vi "Q-Close.vi"(8 "error in":errorcluster, 10 "Queue Type":T1, 11 "Q Name":string) -> (0 "error out":errorcluster)   [LabVIEW 2016]
uses:
  PSDAQEG_Task Queue Type.ctl
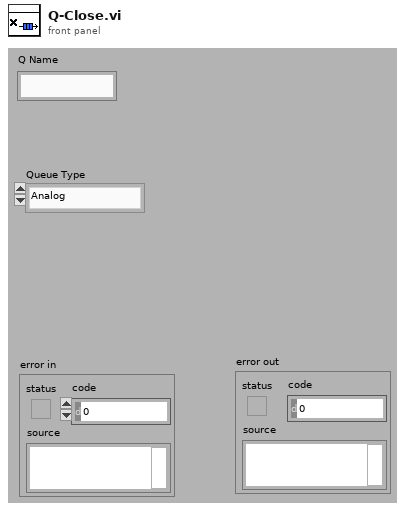
[diagram p1: front panel]
types:
  T1 = typedef "PSDAQEG_Task Queue Type.ctl" = enum16{"Analog", "Digital", "Variant"}
  T2 = cluster{"Analog Data":waveform(dbl)[], "Digital Data":digitalwaveform[], "Variant Data":variant[]}
  T3 = cluster{"max queue size (-1, unlimited)":i32, "Analog Data":waveform(dbl)[]}
  T4 = cluster{"max queue size (-1, unlimited)":i32, "Digital Data":digitalwaveform[]}
  T5 = cluster{"max queue size (-1, unlimited)":i32, "Variant Data":variant[]}
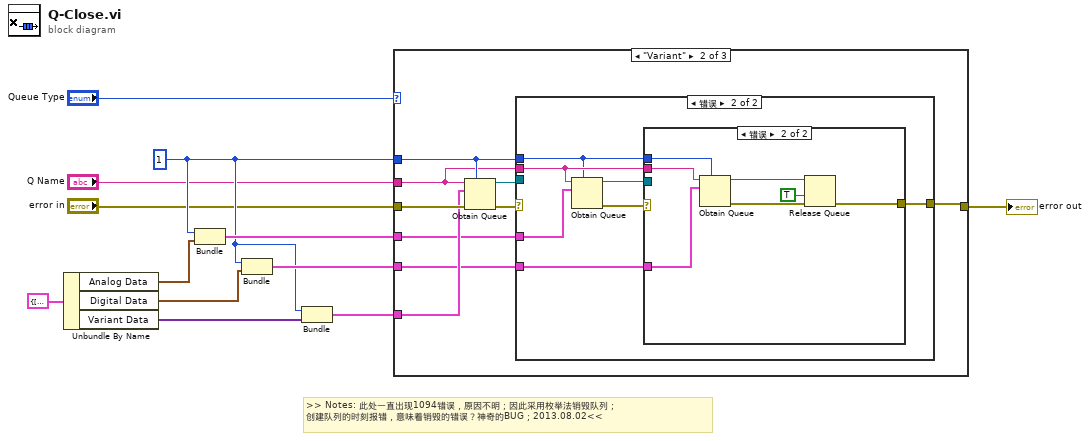
[diagram p0: block diagram]
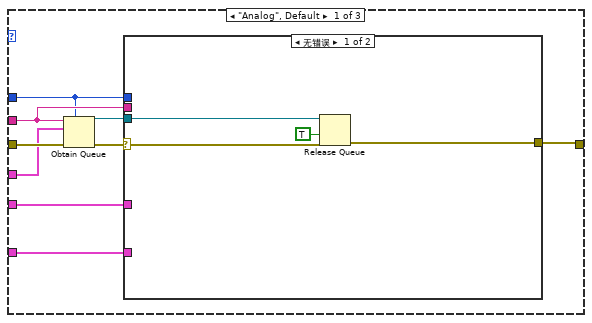
[diagram p2: hidden frame]
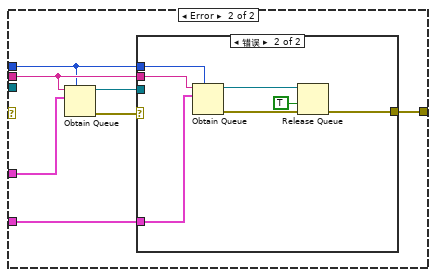
[diagram p3: hidden frame]
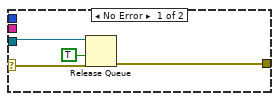
[diagram p4: hidden frame]
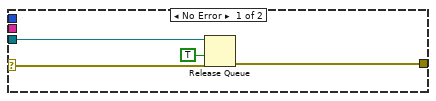
[diagram p5: hidden frame]
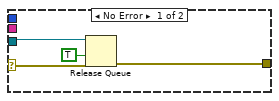
[diagram p6: hidden frame]
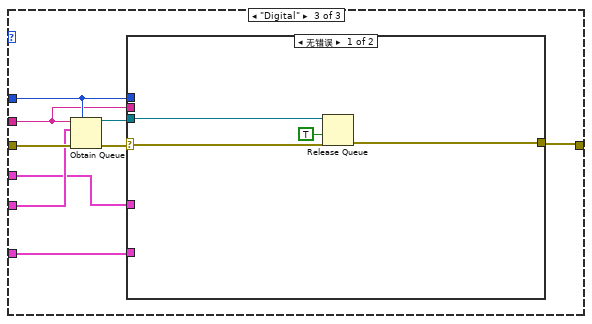
[diagram p7: hidden frame]
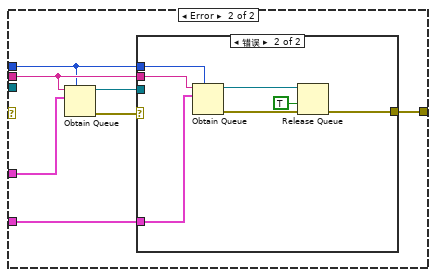
[diagram p8: hidden frame]
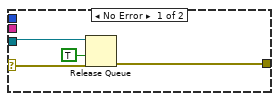
[diagram p9: hidden frame]
diagram:
  w9 = 1 ("max queue size (-1, unlimited)")
  # ">> Notes: 此处一直出现1094错误，原因不明；因此采用枚举法销毁队列；\n创建队列的时刻报错，意味着销毁的错误？神奇的BUG；2013.08.02<<"
  n1 = Unbundle By Name(T2 {"Analog Data"=[], "Digital Data"=[], "Variant Data"=[]} ("Read Data")) -> ("Analog Data"=w3:waveform(dbl)[], "Digital Data"=w2:digitalwaveform[], "Variant Data"=w1:variant[])
  n2 = Bundle("max queue size (-1, unlimited)"=w9, "Analog Data"=w3) -> (w10:T3)  [unwired: 1 in]
  n3 = Bundle("max queue size (-1, unlimited)"=w9, "Digital Data"=w2) -> (w11:T4)  [unwired: 1 in]
  n4 = Bundle("max queue size (-1, unlimited)"=w9, "Variant Data"=w1) -> (w8:T5)  [unwired: 1 in]
  n5 = case shown="\"Variant\"" "Queue Type" {
    tunnel: "Q Name" -> [w16 w46 w78]
    tunnel: "error in" -> [w21 w52 w83]
    tunnel: w9 -> [w15 w47 w79]
    tunnel: w11 -> [w14 w44 w82]
    tunnel: [w18 w48 w80] -> w5
    tunnel: w10 -> [w20 w45 w76]
    tunnel: w8 -> [w13 w51 w75]
    frame "Analog", Default {
      n6 = Obtain Queue(max queue size (-1, unlimited)=w15, name (unnamed)=w16, element data type=w20, error in (no error)=w21) -> (queue out=w19:refnum<queue>, error out=w17:errorcluster)  [unwired: 1 in, 1 out]
      n7 = case shown="无错误" w17 {
        selector: w17 -> [w22 _]
        tunnel: w19 -> [w24 _]
        tunnel: [w23 w29] -> w18
        tunnel: w16 -> [_ w28]
        tunnel: w15 -> [_ w27]
        tunnel: w14 -> [_ w32]
        tunnel: w13 -> [_ w26]
        frame No Error {
          n8 = Release Queue(queue=w24, force destroy? (F)=TRUE, error in (no error)=w22) -> (error out=w23:errorcluster)  [unwired: 2 out]
        }
        frame Error {
          n9 = Obtain Queue(max queue size (-1, unlimited)=w27, name (unnamed)=w28, element data type=w32) -> (queue out=w30:refnum<queue>, error out=w31:errorcluster)  [unwired: 2 in, 1 out]
          n10 = case shown="错误" w31 {
            selector: w31 -> [w34 _]
            tunnel: w30 -> [w35 _]
            tunnel: [w33 w38] -> w29
            tunnel: w28 -> [_ w43]
            tunnel: w27 -> [_ w42]
            tunnel: w26 -> [_ w41]
            frame No Error {
              n11 = Release Queue(queue=w35, force destroy? (F)=TRUE, error in (no error)=w34) -> (error out=w33:errorcluster)  [unwired: 2 out]
            }
            frame Error {
              n12 = Obtain Queue(max queue size (-1, unlimited)=w42, name (unnamed)=w43, element data type=w41) -> (queue out=w37:refnum<queue>, error out=w39:errorcluster)  [unwired: 2 in, 1 out]
              n13 = Release Queue(queue=w37, force destroy? (F)=TRUE, error in (no error)=w39) -> (error out=w38:errorcluster)  [unwired: 2 out]
            }
          }
        }
      }
    }
    frame "Variant" {
      n14 = Obtain Queue(max queue size (-1, unlimited)=w47, name (unnamed)=w46, element data type=w51, error in (no error)=w52) -> (queue out=w49:refnum<queue>, error out=w50:errorcluster)  [unwired: 1 in, 1 out]
      n15 = case shown="错误" w50 {
        selector: w50 -> [w53 _]
        tunnel: w49 -> [w55 _]
        tunnel: [w54 w60] -> w48
        tunnel: w46 -> [_ w59]
        tunnel: w47 -> [_ w58]
        tunnel: w45 -> [_ w63]
        tunnel: w44 -> [_ w57]
        frame No Error {
          n16 = Release Queue(queue=w55, force destroy? (F)=TRUE, error in (no error)=w53) -> (error out=w54:errorcluster)  [unwired: 2 out]
        }
        frame Error {
          n17 = Obtain Queue(max queue size (-1, unlimited)=w58, name (unnamed)=w59, element data type=w63) -> (queue out=w61:refnum<queue>, error out=w62:errorcluster)  [unwired: 2 in, 1 out]
          n18 = case shown="错误" w62 {
            selector: w62 -> [w65 _]
            tunnel: w61 -> [w66 _]
            tunnel: [w64 w69] -> w60
            tunnel: w59 -> [_ w74]
            tunnel: w58 -> [_ w73]
            tunnel: w57 -> [_ w72]
            frame No Error {
              n19 = Release Queue(queue=w66, force destroy? (F)=TRUE, error in (no error)=w65) -> (error out=w64:errorcluster)  [unwired: 2 out]
            }
            frame Error {
              n20 = Obtain Queue(max queue size (-1, unlimited)=w73, name (unnamed)=w74, element data type=w72) -> (queue out=w68:refnum<queue>, error out=w70:errorcluster)  [unwired: 2 in, 1 out]
              n21 = Release Queue(queue=w68, force destroy? (F)=TRUE, error in (no error)=w70) -> (error out=w69:errorcluster)  [unwired: 2 out]
            }
          }
        }
      }
    }
    frame "Digital" {
      n22 = Obtain Queue(max queue size (-1, unlimited)=w79, name (unnamed)=w78, element data type=w82, error in (no error)=w83) -> (queue out=w77:refnum<queue>, error out=w81:errorcluster)  [unwired: 1 in, 1 out]
      n23 = case shown="无错误" w81 {
        selector: w81 -> [w84 _]
        tunnel: w77 -> [w86 _]
        tunnel: [w85 w91] -> w80
        tunnel: w78 -> [_ w90]
        tunnel: w79 -> [_ w89]
        tunnel: w76 -> [_ w94]
        tunnel: w75 -> [_ w88]
        frame No Error {
          n24 = Release Queue(queue=w86, force destroy? (F)=TRUE, error in (no error)=w84) -> (error out=w85:errorcluster)  [unwired: 2 out]
        }
        frame Error {
          n25 = Obtain Queue(max queue size (-1, unlimited)=w89, name (unnamed)=w90, element data type=w94) -> (queue out=w92:refnum<queue>, error out=w93:errorcluster)  [unwired: 2 in, 1 out]
          n26 = case shown="错误" w93 {
            selector: w93 -> [w96 _]
            tunnel: w92 -> [w97 _]
            tunnel: [w95 w100] -> w91
            tunnel: w90 -> [_ w105]
            tunnel: w89 -> [_ w104]
            tunnel: w88 -> [_ w103]
            frame No Error {
              n27 = Release Queue(queue=w97, force destroy? (F)=TRUE, error in (no error)=w96) -> (error out=w95:errorcluster)  [unwired: 2 out]
            }
            frame Error {
              n28 = Obtain Queue(max queue size (-1, unlimited)=w104, name (unnamed)=w105, element data type=w103) -> (queue out=w99:refnum<queue>, error out=w101:errorcluster)  [unwired: 2 in, 1 out]
              n29 = Release Queue(queue=w99, force destroy? (F)=TRUE, error in (no error)=w101) -> (error out=w100:errorcluster)  [unwired: 2 out]
            }
          }
        }
      }
    }
  }
  "error out" <- w5
